vi "Update List Log.vi"(9 "Command to Input":string, 11 "reference":refnum<vi>) -> ()   [LabVIEW 2020]
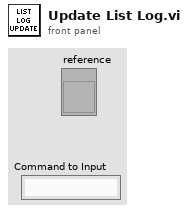
[diagram p1: front panel]
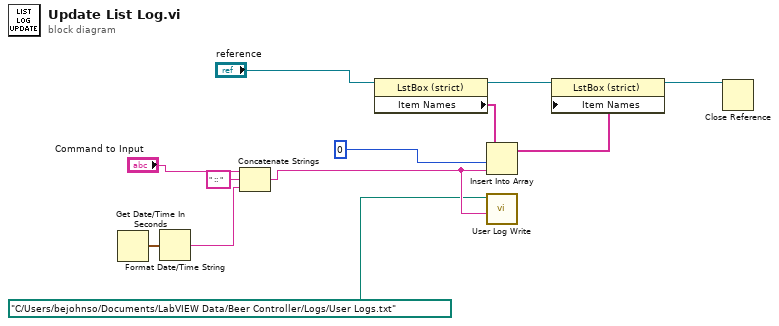
[diagram p0: block diagram]
diagram:
  n1 = Get Date/Time In Seconds() -> (seconds since 1Jan1904=w6:timestamp)
  n2 = Format Date/Time String(seconds (now)=w6) -> (date/time string=w4:string)  [unwired: 2 in]
  n3 = Concatenate Strings("Command to Input", " :: " ("string"), w4) -> (w2:string)
  n4 = property class="LstBox (strict)"(reference="reference") -> (reference out=w9:refnum<vi>, "Item Names"=w12:string[])  [unwired: 1 in, 1 out]
  n5 = Insert Into Array(array=w12, index=0, new element=w2) -> (w11:string[])
  n6 = call "User Log Write.vi"("User Info to Write"=w2, "File Location of User Logs"=path "C:/Users/bejohnso/Documents/LabVIEW Data/Beer Controller/Logs/User Logs.txt") -> ()  [unwired: 9 in, 1 out]
  n7 = property class="LstBox (strict)"(reference=w9, "Item Names"=w11) -> (reference out=w8:refnum<vi>)  [unwired: 1 in, 1 out]
  n8 = Close Reference(reference=w8) -> ()  [unwired: 1 in, 1 out]
